vi "GetControlReferenceTypesList.vi"(8 "error in (no error)":errorcluster, 11 "ByteGSWebAPI-V0 in":refnum<class "ByteGSWebAPI-V0.lvclass">) -> (0 "error out":errorcluster, 2 "ControlReferenceTypesList":T1, 3 "ByteGSWebAPI-V0 out":refnum<class "ByteGSWebAPI-V0.lvclass">)   [LabVIEW 2019, in "ByteGSWebAPI.lvlib" / "ByteGSWebAPI-V0.lvclass"]
doc: "Richiesta di GET di tutti i control reference (ID: \" \")"
uses:
  ByteGSWebAPI-V0.lvclass
  Cntrls/MultipleControlReferenceType.ctl
  Cntrls/SingleControlReferenceType.ctl
  54c15d21-1fd3-4ea8-80e2-c69b0da6434b.vi
  <vilib>/JDP Science/JSONtext/JSON text to Variant.vi
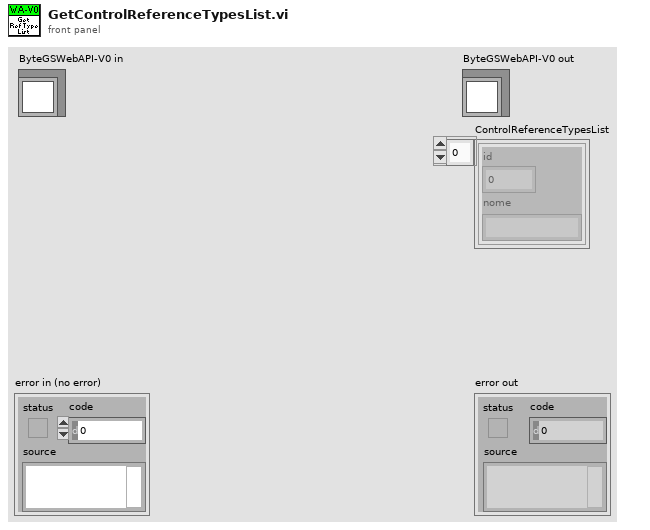
[diagram p1: front panel]
types:
  T1 = typedef "ByteGSWebAPI.lvlib/ByteGSWebAPI-V0.lvclass/MultipleControlReferenceType.ctl" = T2[]
  T2 = typedef "ByteGSWebAPI.lvlib/ByteGSWebAPI-V0.lvclass/SingleControlReferenceType.ctl" = cluster{"id":i32, "nome":string}
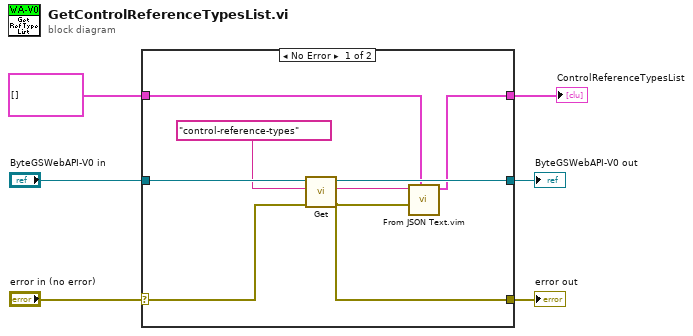
[diagram p0: block diagram]
diagram:
  n1 = case shown="No Error" "error in (no error)" {
    selector: "error in (no error)" -> [w11 w17]
    tunnel: [w9 w17] -> w5
    tunnel: [w13 w16] -> w3
    tunnel: "ByteGSWebAPI-V0 in" -> [w14 w16]
    tunnel: T1 [] ("MultipleControlReferenceType") -> [w8 w15]
    tunnel: [w7 w15] -> w1
    frame No Error {
      n2 = call "Get.vi"("error in (no error)"=w11, "Request"="control-reference-types" ("Parameter"), "ByteGSWebAPI-V0 in"=w14) -> ("error out"=w9:errorcluster, "body"=w10:string, "ByteGSWebAPI-V0 out"=w13:refnum<class "ByteGSWebAPI-V0.lvclass">)  [unwired: 5 in, 1 out]
      n3 = call "From JSON Text.vim"("Data Type and Default Value"=w8, "error in (no error)"=w9, "JSON"=w10) -> ("Data out"=w7:T1)  [unwired: 7 in, 1 out]
    }
    frame Error {
    }
  }
  "error out" <- w5
  "ByteGSWebAPI-V0 out" <- w3
  "ControlReferenceTypesList" <- w1
